vi "CSTK_Icon_Creator_Insert_TitleBGColor.vi"(7 "LOGO":string, 8 "error in (no error)":errorcluster, 9 "标题背景色":u32(colorbox), 11 "图片输入":picture) -> (0 "error out":errorcluster, 3 "图片输出":picture)   [LabVIEW 2015, in "CSTK_Icon Creator.lvlib"]
uses:
  CSTK_Icon Creator.lvlib
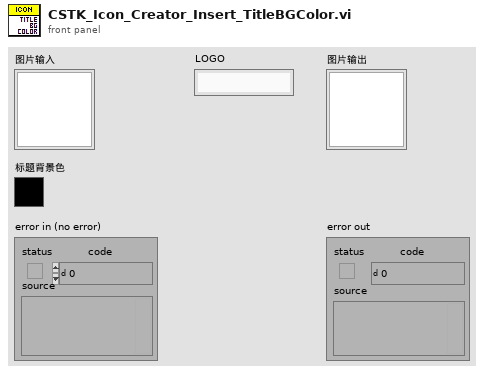
[diagram p1: front panel]
types:
  T1 = cluster{"left":i16, "top":i16, "right":i16, "bottom":i16}
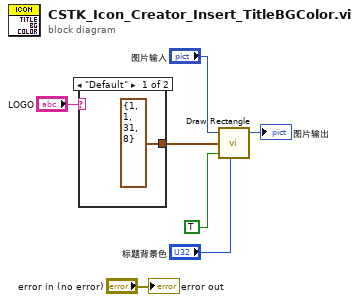
[diagram p0: block diagram]
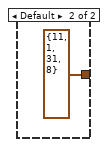
[diagram p2: hidden frame]
diagram:
  n1 = case shown="\"Default\"" "LOGO" {
    tunnel: [T1 {"left"=1, "top"=1, "right"=31, "bottom"=8} ("rect") T1 {"left"=11, "top"=1, "right"=31, "bottom"=8} ("rect")] -> w2
    frame "Default" {
    }
    frame Default {
    }
  }
  n2 = call <vilib>:"Draw Rectangle.vi"("picture"="图片输入", "rect"=w2, "fill?(F)"=TRUE, "color(black)"="标题背景色") -> ("new picture"=→"图片输出":picture)  [unwired: 5 in]
  "error out" <- "error in (no error)"
